vi "get supported types.vi"(8 "error in":errorcluster, 11 "fixed module parent implementation configuration in":refnum<class "fixed channel configuration.lvclass">) -> (0 "error out":errorcluster, 2 "supported types":T1[](array[typedef]), 3 "fixed module parent implementation configuration out":refnum<class "fixed channel configuration.lvclass">)   [LabVIEW 2013, in "fixed channel configuration.lvclass"]
doc: "Provides an interface for determining the targets supported by a given configuration/runtime class pairing. This should be overridden by any useful child class."
uses:
  fixed channel configuration.lvclass
  <vilib>/NI/Tag Bus/tag/Data Type.ctl
  fixed channel configuration.lvclass/fixed channel configuration.ctl
  <vilib>/NI/Tag Bus/tag/tag descriptor.lvclass/tag descriptor.ctl
  <vilib>/NI/Tag Bus/tag/tag descriptor.lvclass
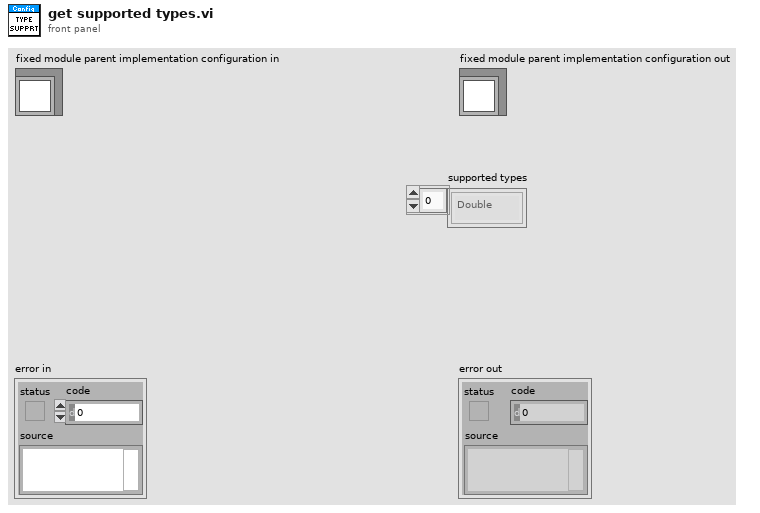
[diagram p1: front panel]
types:
  T1 = typedef "tag bus.lvlib/tag descriptor.lvclass/Data Type.ctl" = enum16{"Double", "Single", "I64", "I32", "I16", "I8", "U64", "U32", "U16", "U8", "Boolean", "String", "Array of Double", "Array of Single", "Array of I64", "Array of I32", "Array of I16", "Array of I8", "Array of U64", "Array of U32", "Array of U16", "Array of U8", "Array of Boolean", "Array of String"}
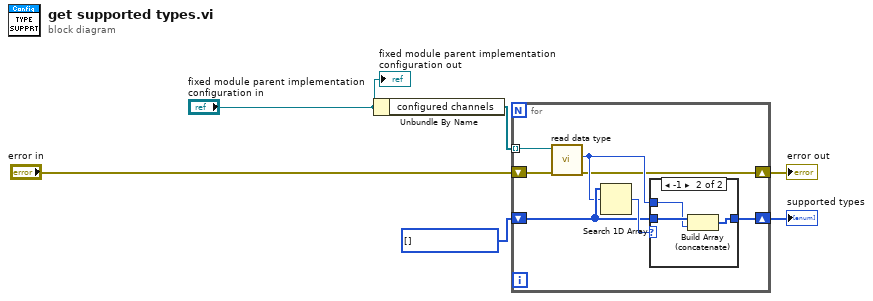
[diagram p0: block diagram]
diagram:
  w4 = T1[] [] items=["Double", "Single", "I64", "I32", "I16", "I8", "U64", "U32", "U16", "U8", "Boolean", "String", "Array of Double", "Array of Single", "Array of I64", "Array of I32", "Array of I16", "Array of I8", "Array of U64", "Array of U32", "Array of U16", "Array of U8", "Array of Boolean", "Array of String"]
  n1 = Unbundle By Name("fixed module parent implementation configuration in") -> ("configured channels"=w5:refnum<class "TBM channel.lvclass">[])
  n2 = for {
    tunnel: w5 -> [w13] mode=indexing
    shift-right: [w9] -> w3
    shift-left: w4 -> [w11]
    shift-right: [w7] -> w1
    shift-left: "error in" -> [w8]
    n3 = call <vilib>:"read data type.vi"("error in"=w8, "system tag in"=w13) -> ("error out"=w7:errorcluster, "data type"=w10:T1)  [unwired: 7 in, 1 out]
    n4 = Search 1D Array(1D array=w11, element=w10) -> (index of element=w12:i32)  [unwired: 1 in]
    n5 = case shown="-1" w12 {
      tunnel: w11 -> [w14 w17]
      tunnel: w10 -> [_ w16]
      tunnel: [w14 w15] -> w9
      frame Default {
      }
      frame -1 {
        n6 = Build Array (concatenate)(w17, w16) -> (w15:T1[])
      }
    }
  }
  "error out" <- w1
  "supported types" <- w3
  "fixed module parent implementation configuration out" <- "fixed module parent implementation configuration in"
